vi "StateQ.vi"(4 "QueueCommand":T3, 5 "error in (no error)":errorcluster, 8 "output cluster":T1) -> (0 "error out":errorcluster, 3 "queue out":refnum<queue>)   [LabVIEW 2020]
doc: "*-----------------------------------------------------\n* Author: SWatts\n*\n* VI Description: Sends Transitions to Wait for Transition\n* \n*\n* Error handling: All errors passed out\n*\n* Pre-condition: \n*\n* Post-condition: None\n*\n* Revision History:\n*\n* Rev Date Author Description \n* 01 30/04/2014 SWatts First issue\n*\n*-----------------------------------------------------"
uses:
  Controls/QueueCommand.ctl
  Controls/StateMessage.ctl
  Controls/Transition.ctl
panel:
  # "Input"
  # "Output"
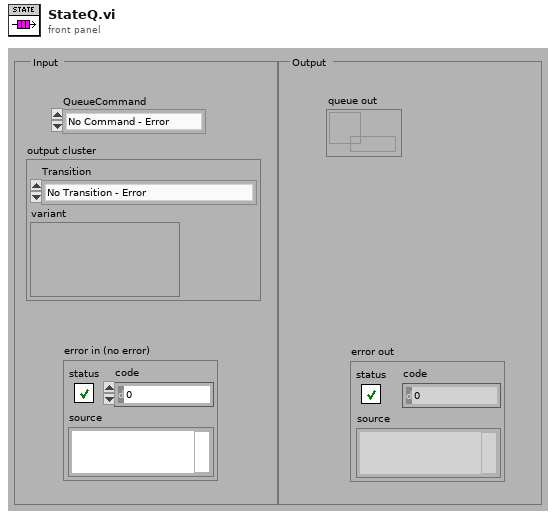
[diagram p1: front panel]
types:
  T1 = typedef "StateMessage.ctl" = cluster{"Transition":T2, "variant":variant}
  T2 = typedef "Transition.ctl" = enum16{"No Transition - Error", "Initialise", "Connected", "Timed Out", "Disconnected", "Message Rxd", "Generate Error", "Start", "Stop", "Exit"}
  T3 = typedef "QueueCommand.ctl" = enum16{"No Command - Error", "Initialise", "Add to Bottom", "Add To Top", "Get Ref", "Close"}
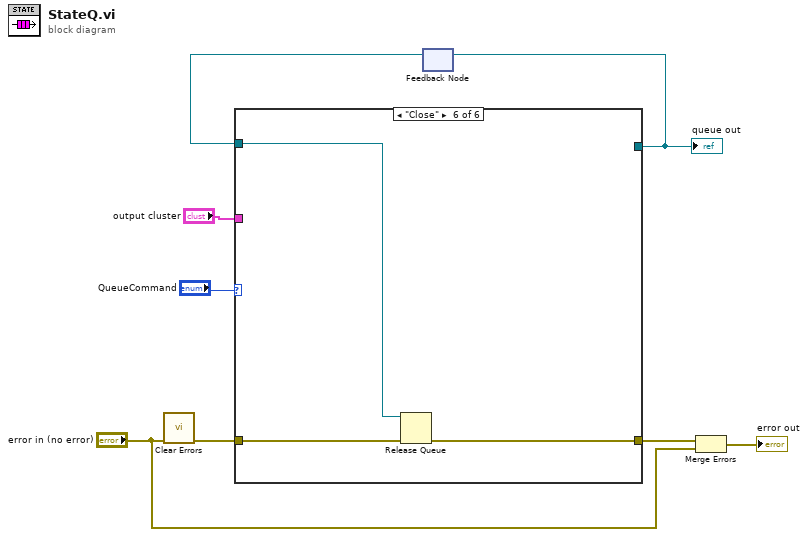
[diagram p0: block diagram]
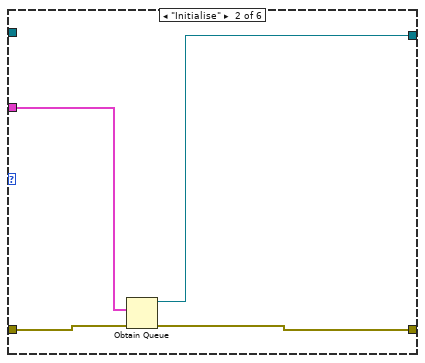
[diagram p3: hidden frame]
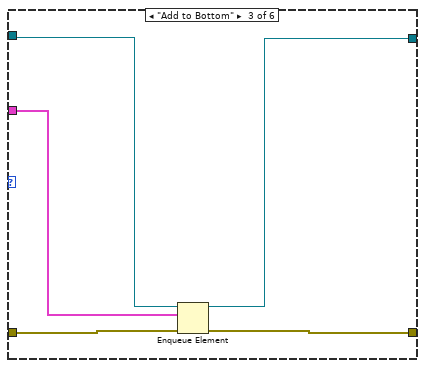
[diagram p4: hidden frame]
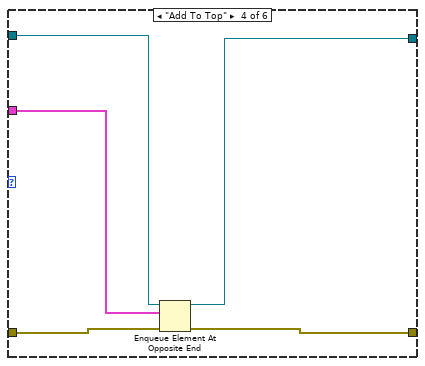
[diagram p5: hidden frame]
diagram:
  n1 = call <vilib>:"Clear Errors.vi"("error in (no error)"="error in (no error)") -> ("error out"=w1:errorcluster)  [unwired: 5 in, 1 out]
  n2 = feedback #1() -> (w5:refnum<queue>)  [unwired: 1 in]
  n3 = case shown="\"Close\"" "QueueCommand" {
    tunnel: "output cluster" -> [_ w14 w15 w20 _ _]
    tunnel: [w10 w13 w16 w22 w26 _] -> w6
    tunnel: w5 -> [w10 _ w17 w21 w26 w27]
    tunnel: w1 -> [w9 w12 w19 w24 w25 w29]
    tunnel: [w9 w11 w18 w23 w25 w28] -> w4
    frame "No Command - Error", Default {
    }
    frame "Initialise" {
      n4 = Obtain Queue(element data type=w14, error in (no error)=w12) -> (queue out=w13:refnum<queue>, error out=w11:errorcluster)  [unwired: 3 in, 1 out]
    }
    frame "Add to Bottom" {
      n5 = Enqueue Element(queue=w17, element=w15, error in (no error)=w19) -> (queue out=w16:refnum<queue>, error out=w18:errorcluster)  [unwired: 1 in, 1 out]
    }
    frame "Add To Top" {
      n6 = Enqueue Element At Opposite End(queue=w21, element=w20, error in (no error)=w24) -> (queue out=w22:refnum<queue>, error out=w23:errorcluster)  [unwired: 1 in, 1 out]
    }
    frame "Get Ref" {
    }
    frame "Close" {
      n7 = Release Queue(queue=w27, error in (no error)=w29) -> (error out=w28:errorcluster)  [unwired: 1 in, 2 out]
    }
  }
  "queue out" <- w6
  n8 = feedback-in #1(w6) -> ()
  n9 = Merge Errors(w4, "error in (no error)") -> (→"error out":errorcluster)
